vi "Write Reader SerialNO.vi"(0 "COM":refnum<visa-resource-name>, 1 "Timeout (ms)":u32=500, 7 "Address":string="01", 11 "error in (no error)":errorcluster) -> (4 "COM OUT":refnum<visa-resource-name>, 6 "Reader SN":string, 15 "error out":errorcluster)   [LabVIEW 2020, in "Reader.lvlib"]
uses:
  Reader.lvlib
panel:
  in  "SerialNo":string
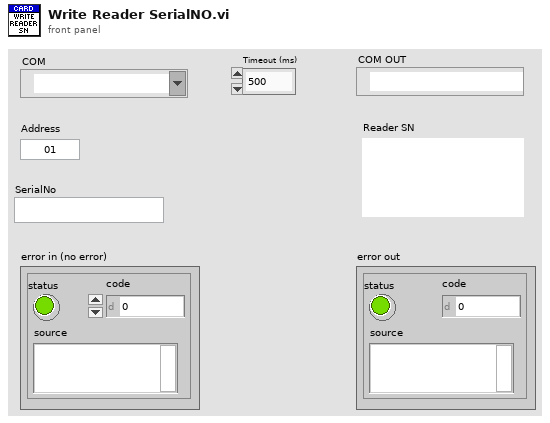
[diagram p1: front panel]
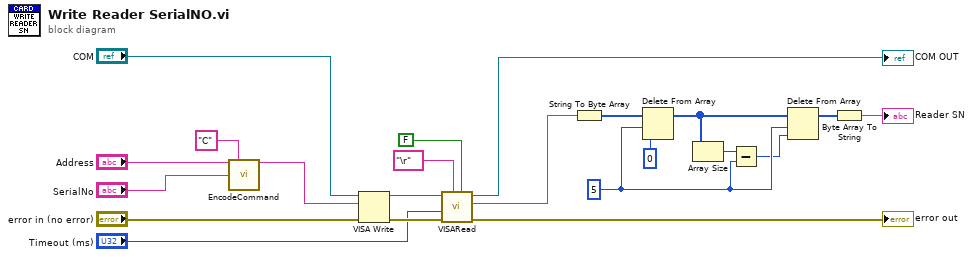
[diagram p0: block diagram]
diagram:
  w6 = 5 ("length (len. of substring)")
  n1 = call "EncodeCommand.vi"("Address"="Address", "Function"="C", "Data"="SerialNo") -> ("Command String"=w17:string)  [unwired: 11 in, 1 out]
  n2 = VISA Write(VISA resource name="COM", write buffer=w17, error in (no error)="error in (no error)") -> (VISA resource name out=w19:refnum<visa-resource-name>, error out=w18:errorcluster)  [unwired: 1 out]
  n3 = call "VISARead.vi"("Delete Termination Char (False)"=FALSE, "Termination Char (blank)"="\r" ("Read regular"), "error in (no error)"=w18, "Timeout (ms)"="Timeout (ms)", "Resource in"=w19) -> ("error out"=→"error out":errorcluster, "Read Char"=w3:string, "Resource out"=→"COM OUT":refnum<visa-resource-name>)  [unwired: 4 in]
  n4 = String To Byte Array(string=w3) -> (unsigned byte array=w10:u8[])
  n5 = Delete From Array(array=w10, length=w6, index=0) -> (array with subset deleted=w8:u8[])  [unwired: 1 out]
  n6 = Array Size(array=w8) -> (size(s)=w7:i32)
  n7 = Subtract(x=w7, y=w6) -> (x-y=w5:i32)
  n8 = Delete From Array(array=w8, length=w6, index=w5) -> (array with subset deleted=w4:u8[])  [unwired: 1 out]
  n9 = Byte Array To String(unsigned byte array=w4) -> (string=→"Reader SN":string)
